vi "Logger Main.vi"(0 "State":string, 11 "error in (no error)":errorcluster) -> (15 "error out":errorcluster)   [LabVIEW 2021, in "Error Logger.lvlib"]
uses:
  Error Logger.lvlib
  <vilib>/Utility/file.llb/Read Delimited Spreadsheet (string).vi
  <vilib>/Utility/file.llb/Write Delimited Spreadsheet (string).vi
  Converter/Path Functions/Path Functions.lvlib
  Converter/Converter Reusables/Converter Reusables.lvlib
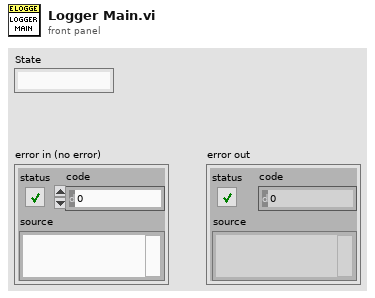
[diagram p1: front panel]
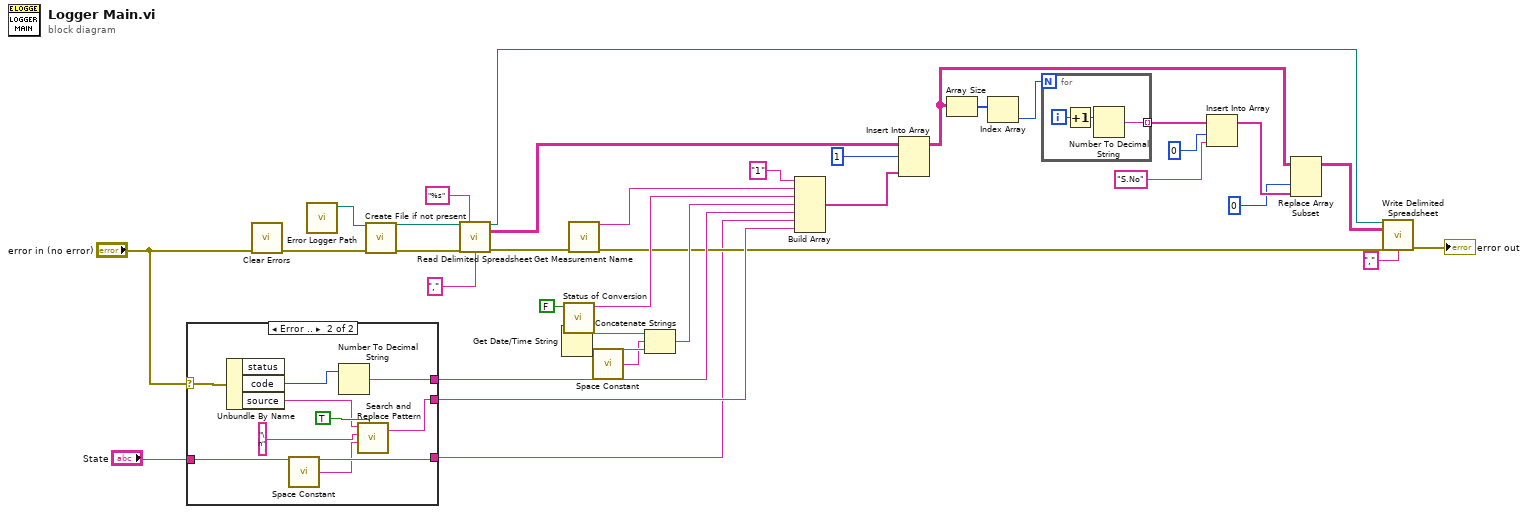
[diagram p0: block diagram]
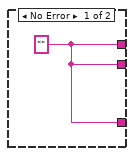
[diagram p2: hidden frame]
diagram:
  n1 = case shown="Error .." "error in (no error)" {
    selector: "error in (no error)" -> [_ w46]
    tunnel: [w37 w44] -> w24
    tunnel: [w37 w38] -> w23
    tunnel: [w37 w43] -> w15
    tunnel: "State" -> [_ w43]
    frame No Error {
      w37 = ""
    }
    frame Error {
      n2 = Unbundle By Name(w46) -> ("code"=w45:i32, "source"=w41:string)  [unwired: 1 out]
      n3 = call <vilib>:"Space Constant.vi"() -> ("String"=w39:string)
      n4 = Number To Decimal String(number=w45) -> (decimal integer string=w44:string)  [unwired: 1 in]
      n5 = call <vilib>:"Search and Replace Pattern.vi"("string"=w41, "regular expression (\"\")"="\n" ("regular expression (\"\")"), "replace string (\"\")"=w39, "replace all? (F)"=TRUE) -> ("result string"=w38:string)  [unwired: 1 in, 1 out]
    }
  }
  n6 = call <vilib>:"Clear Errors.vi"("error in (no error)"="error in (no error)") -> ("error out"=w26:errorcluster)  [unwired: 5 in, 1 out]
  n7 = call "Error Logger Path.vi"() -> ("Error Logger Path"=w36:path)  [unwired: 7 in]
  n8 = call "Create File if not present.vi"("Error Logger Path"=w36, "error in (no error)"=w26) -> ("Duplicate Path"=w34:path, "error out"=w35:errorcluster)  [unwired: 12 in]
  n9 = call-poly <vilib>:"Read Delimited Spreadsheet.vi"("file path (dialog if empty)"=w34, "format (%s)"="%s" ("format (%.3f)"), "error in (no error)"=w35, "delimiter (\\t)"="," ("delimiter (\\t)")) -> ("new file path (Not A Path if cancelled)"=w19:path, "all rows"=w22:string[][], "error out"=w30:errorcluster)  [unwired: 6 in, 3 out]
  n10 = Get Date/Time String() -> (date string=w28:string, time string=w2:string)  [unwired: 3 in]
  n11 = call "Status of Conversion.vi"("Pass?T"=FALSE) -> ("Status"=w29:string)  [unwired: 6 in]
  n12 = call "Get Measurement Name.vi"("error in (no error)"=w30) -> ("Name Out"=w31:string, "error out"=w20:errorcluster)  [unwired: 13 in]
  n13 = call <vilib>:"Space Constant.vi"() -> ("String"=w1:string)
  n14 = Concatenate Strings(w28, w1, w2) -> (w27:string)
  n15 = Build Array("1" ("element"), w31, w29, w27, w24, w15, w23) -> (w13:string[])
  n16 = Insert Into Array(array=w22, index (row)=1, new element=w13) -> (w6:string[][])  [unwired: 1 in]
  n17 = Array Size(array=w6) -> (size(s)=w11:i32[])
  n18 = Index Array(array=w11) -> (element=w10:i32)  [unwired: 1 in]
  n19 = for {
    N: w10 -> [_]
    tunnel: [w48] -> w9 mode=indexing
    i -> [w49]
    n20 = Increment(x=w49) -> (x+1=w47:i32)
    n21 = Number To Decimal String(number=w47) -> (decimal integer string=w48:string)  [unwired: 1 in]
  }
  n22 = Insert Into Array(array=w9, index=0, new element="S.No" ("new element/subarray")) -> (w4:string[])
  n23 = Replace Array Subset(array=w6, new element=w4, index (col)=0 ("disabled index (col)")) -> (w5:string[][])  [unwired: 1 in]
  n24 = call-poly <vilib>:"Write Delimited Spreadsheet.vi"("file path (dialog if empty)"=w19, "2D data"=w5, "error in (no error)"=w20, "delimiter (\\t)"="," ("delimiter (\\t)")) -> ("error out"=→"error out":errorcluster)  [unwired: 10 in, 1 out]
